vi "GetQR.vi"(8 "error in":errorcluster, 9 "STOP":bool, 10 "Image In":T2, 11 "Session In":T1) -> (0 "error out":errorcluster, 2 "QR_CODE":string, 3 "Image Out":T2(plugin-control))   [LabVIEW 2018]
uses:
  <vilib>/vision/Image Controls.llb/IMAQ Image.ctl
  <vilib>/userdefined/High Color/IMAQdx.ctl
  <vilib>/vision/NI_Vision_Development_Module.lvlib
  <vilib>/vision/driver/NI_Vision_Acquisition_Software.lvlib
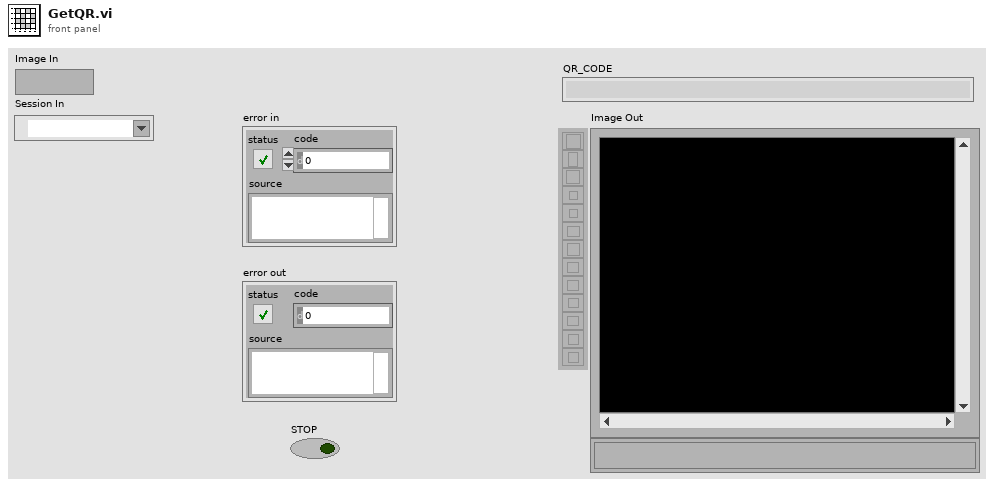
[diagram p1: front panel]
types:
  T1 = typedef "IMAQdx.ctl" = refnum<k21>
  T2 = typedef "IMAQ Image.ctl" = refnum<image>
  T3 = cluster{"Matrix Dimensions (cells)":i32, "Barcode Polarity":i32, "Mirror Mode":i32, "QR Model":i32}
  T4 = cluster{"Rotation Mode":enum32{"Unlimited", "0 Degrees", "90 Degrees", "180 Degrees", "270 Degrees"}, "Skip Location?":bool, "Edge Threshold":u32, "Demodulation Mode":i32, "Cell Sample Size":i32, "Cell Filter Mode":i32, "Skew Degrees Allowed":u32}
  T5 = cluster{"Global Rectangle":i32[], "Contours":cluster{"ID":enum32{"External", "Internal"}, "Type":u32, "Coordinates":i32[]}[]}
  T6 = typedef "QR Code Report.ctl" = cluster{"Found?":bool, "Data":string, "Bounding Box":cluster{"x":sgl, "y":sgl}[], "Errors Corrected":u32, "Dimensions (Rows/Cols)":u32, "Version":u32, "QR Model":T7, "Stream Mode":T8, "Barcode Polarity":T9, "Mirrored?":bool, "Append Stream Position":u32, "Size of Append Stream":u32, "First EAN-128 ID":i32, "First Alternate Language ID":i32, "Append Stream ID":u32, "Minimum Edge Strength":u32, "Demodulation Mode":T10, "Cell Sample Size":T11, "Cell Filter Mode":T12}
  T7 = typedef "QR Code Model Type.ctl" = i32
  T8 = typedef "QR Code Stream Mode Type.ctl" = i32
  T9 = typedef "Data Matrix Polarity.ctl" = i32
  T10 = typedef "Demodulation Mode.ctl" = i32
  T11 = typedef "Cell Sample Size.ctl" = i32
  T12 = typedef "Cell Filter Mode.ctl" = i32
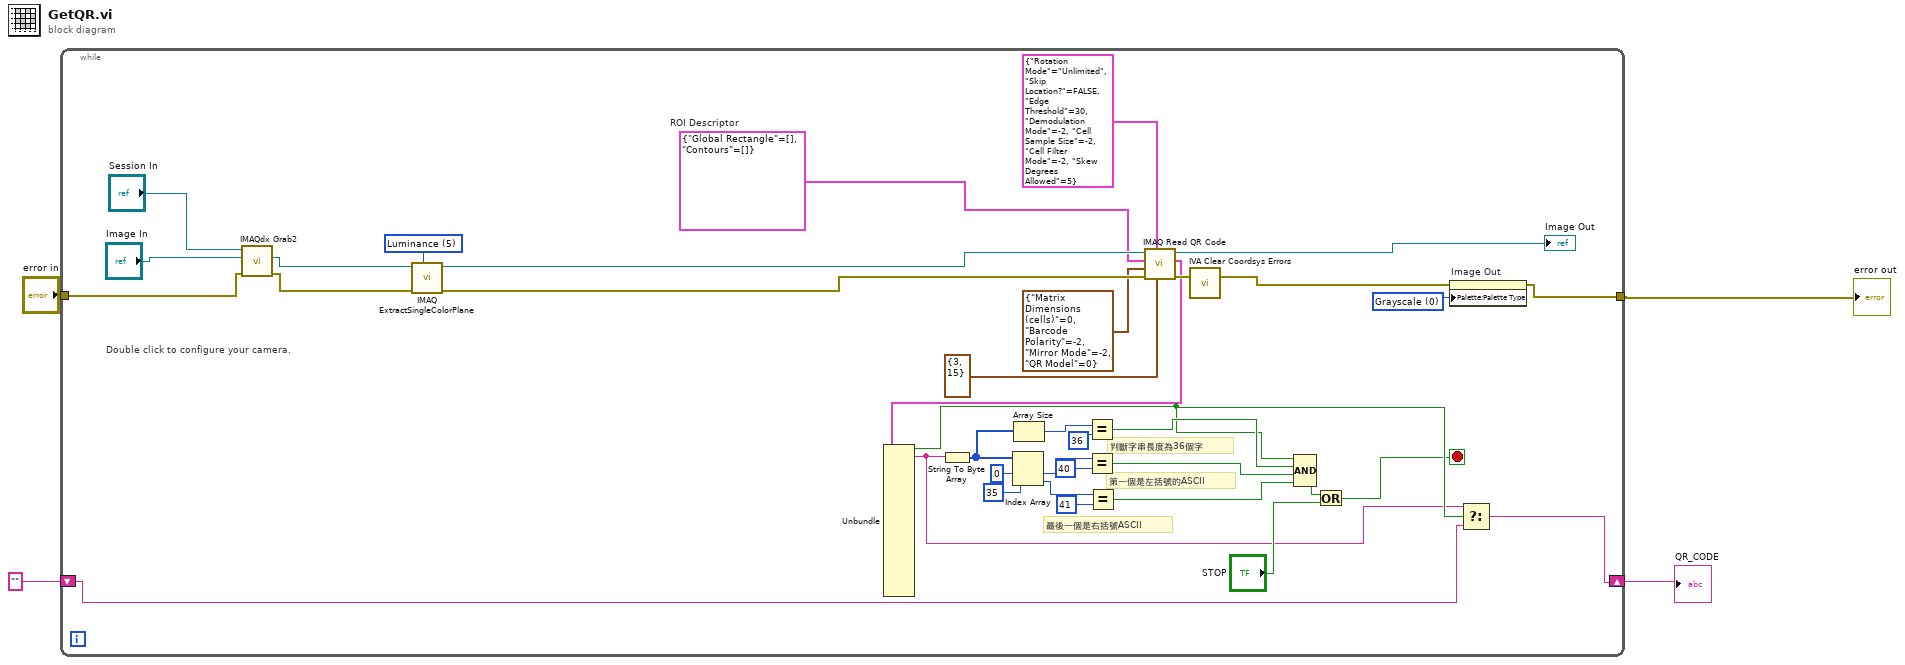
[diagram p0: block diagram]
diagram:
  n1 = while {
    tunnel: "error in" -> [w7]
    tunnel: [w30] -> w1
    shift-right: [w11] -> w2
    shift-left: "" -> [w12]
    stop <- w10 stop-if-true
    w31 = u32 0 items=["Grayscale", "Binary", "Gradient", "Rainbow", "Temperature", "User Defined", "Binary 16 Bit", "Gradient 16 Bit", "Rainbow 16 Bit", "Temperature 16 Bit", "User Defined 16 Bit"] ("Palette Type")
    w35 = T5 {"Global Rectangle"=[], "Contours"=[]}  # ROI Descriptor
    w41 = 5 items=["Red", "Green", "Blue", "Hue", "Saturation", "Luminance", "Value", "Intensity"] ("Color Plane")
    # "最後一個是右括號ASCII"
    # "第一個是左括號的ASCII"
    # "判斷字串長度為36個字"
    # "Double click to configure your camera."
    n2 = call <vilib>:"IMAQdx Grab2.vi"("error in"=w7, "Image In"="Image In", "Session In"="Session In") -> ("error out"=w6:errorcluster, "Image Out"=w5:T2)  [unwired: 5 in, 2 out]
    n3 = call "IMAQ ExtractSingleColorPlane"("Color Plane"=w41, "error in (no error)"=w6, "Image Src"=w5) -> ("error out"=w40:errorcluster, "Image Dst Out"=w39:T2)  [unwired: 1 in, 6 out]
    n4 = call "IMAQ Read QR Code"("QR Code Cell Size (pixels)"=cluster{"Minimum Size":u32, "Maximum Size":u32} {"Minimum Size"=3, "Maximum Size"=15}, "QR Search Options"=T4 {"Rotation Mode"=enum."Unlimited", "Skip Location?"=FALSE, "Edge Threshold"=30, "Demodulation Mode"=-2, "Cell Sample Size"=-2, "Cell Filter Mode"=-2, "Skew Degrees Allowed"=5}, "error in (no error)"=w40, "QR Description Options"=T3 {"Matrix Dimensions (cells)"=0, "Barcode Polarity"=-2, "Mirror Mode"=-2, "QR Model"=0}, "ROI Descriptor"=w35, "Image"=w39) -> ("error out"=w34:errorcluster, "QR Code Report"=w29:T6, "Image (duplicate)"=→"Image Out":T2)  [unwired: 1 in, 2 out]
    n5 = Unbundle(w29) -> ("Found?"=w14:bool, "Data"=w13:string)  [unwired: 17 out]
    n6 = String To Byte Array(string=w13) -> (unsigned byte array=w17:u8[])
    n7 = Index Array(array=w17, index #1=0 ("index"), index #2=35 ("index")) -> (element #1=w24:u8, element #2=w23:u8)
    n8 = Array Size(array=w17) -> (size(s)=w28:i32)
    n9 = Equal?(x=w28, y=36) -> (x = y?=w20:bool)
    n10 = Equal?(x=w24, y=u8 40) -> (x = y?=w19:bool)
    n11 = Equal?(x=w23, y=u8 41) -> (x = y?=w18:bool)
    n12 = call <vilib>:"IVA Clear Coordsys Errors.vi"("error in (no error)"=w34) -> ("error out"=w33:errorcluster)  [unwired: 10 in]
    n13 = Compound Arithmetic op=AND(w14, w20, w19, w18) -> (w16:bool)
    n14 = Or(x=w16, y="STOP") -> (x .or. y?=w10:bool)
    n15 = property on="Image Out" class="ImageControl"(error in=w33, "Palette:Palette Type"=w31) -> (error out=w30:errorcluster)  [unwired: 1 in, 1 out]
    n16 = Select(t=w13, s=w14, f=w12) -> (s? t:f=w11:string)
  }
  "error out" <- w1
  "QR_CODE" <- w2
